vi "Read_Website_HTML-modified v01.vi"(5 "URL":string) -> (1 "length":i32, 2 "HTML as string":string)   [LabVIEW 2013]
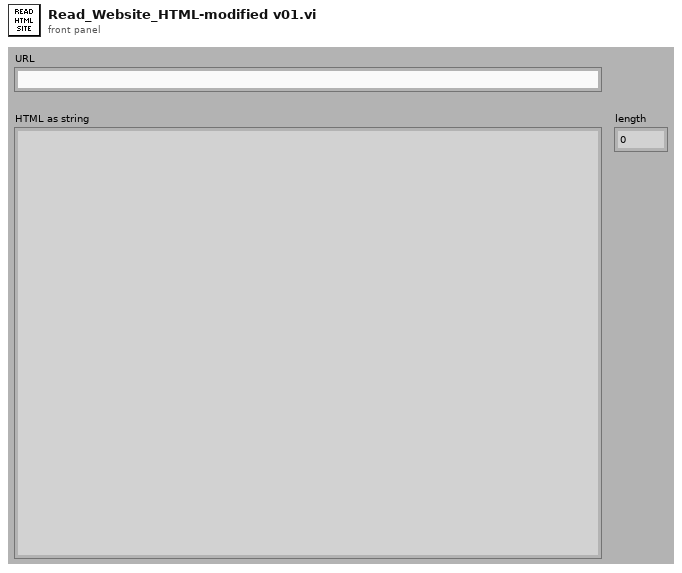
[diagram p1: front panel]
types:
  T1 = enum16{"Read", "Write", "ReadWrite", "BufferedRead", "BufferedReadWrite"}
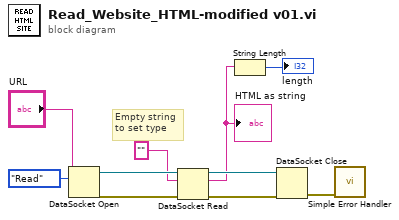
[diagram p0: block diagram]
diagram:
  # "Empty string\nto set type"
  n1 = DataSocket Open(10:T1."Read" ("mode"), 11:"URL") -> (0:w7:errorcluster, 3:w10:refnum<k13>)  [unwired: 2 in]
  n2 = DataSocket Read(8:w7, 10:"", 11:w10) -> (0:w8:errorcluster, 2:w2:string, 3:w9:refnum<k13>)  [unwired: 2 in, 4 out]
  "HTML as string" <- w2
  n3 = String Length(string=w2) -> (length=→"length":i32)
  n4 = DataSocket Close(8:w8, 11:w9) -> (0:w3:errorcluster)  [unwired: 1 in, 1 out]
  n5 = call <vilib>:"Simple Error Handler.vi"("error in (no error)"=w3) -> ()  [unwired: 4 in, 5 out]
